vi "wherestheline.vi"(0 "SCin":u16=15000 min=10240 max=19650 step=100, 1 "S1in":u16=15000 min=10240 max=19650 step=100, 2 "S2in":u16=15000 min=10240 max=19650 step=100, 3 "S3in":u16=15000 min=10240 max=19650 step=100, 4 "S4in":u16=15000 min=10240 max=19650 step=100, 5 "S5in":u16=15000 min=10240 max=19650 step=100, 7 "last error":dbl=15000.0 min=10240.0 max=19650.0 step=100.0) -> (19 "SC":bool, 20 "error":dbl, 21 "line found":bool, 22 "really lost":bool, 23 "S1":bool, 24 "S2":bool, 25 "S3":bool, 26 "S4":bool, 27 "S5":bool)   [LabVIEW 2011]
panel:
  out "orS4":bool
  out "orS2":bool
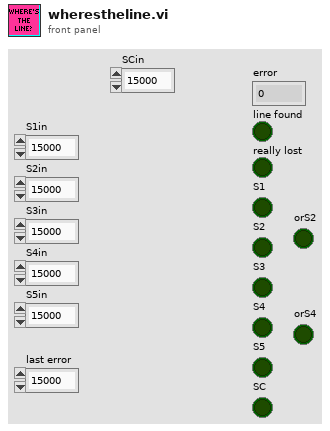
[diagram p1: front panel]
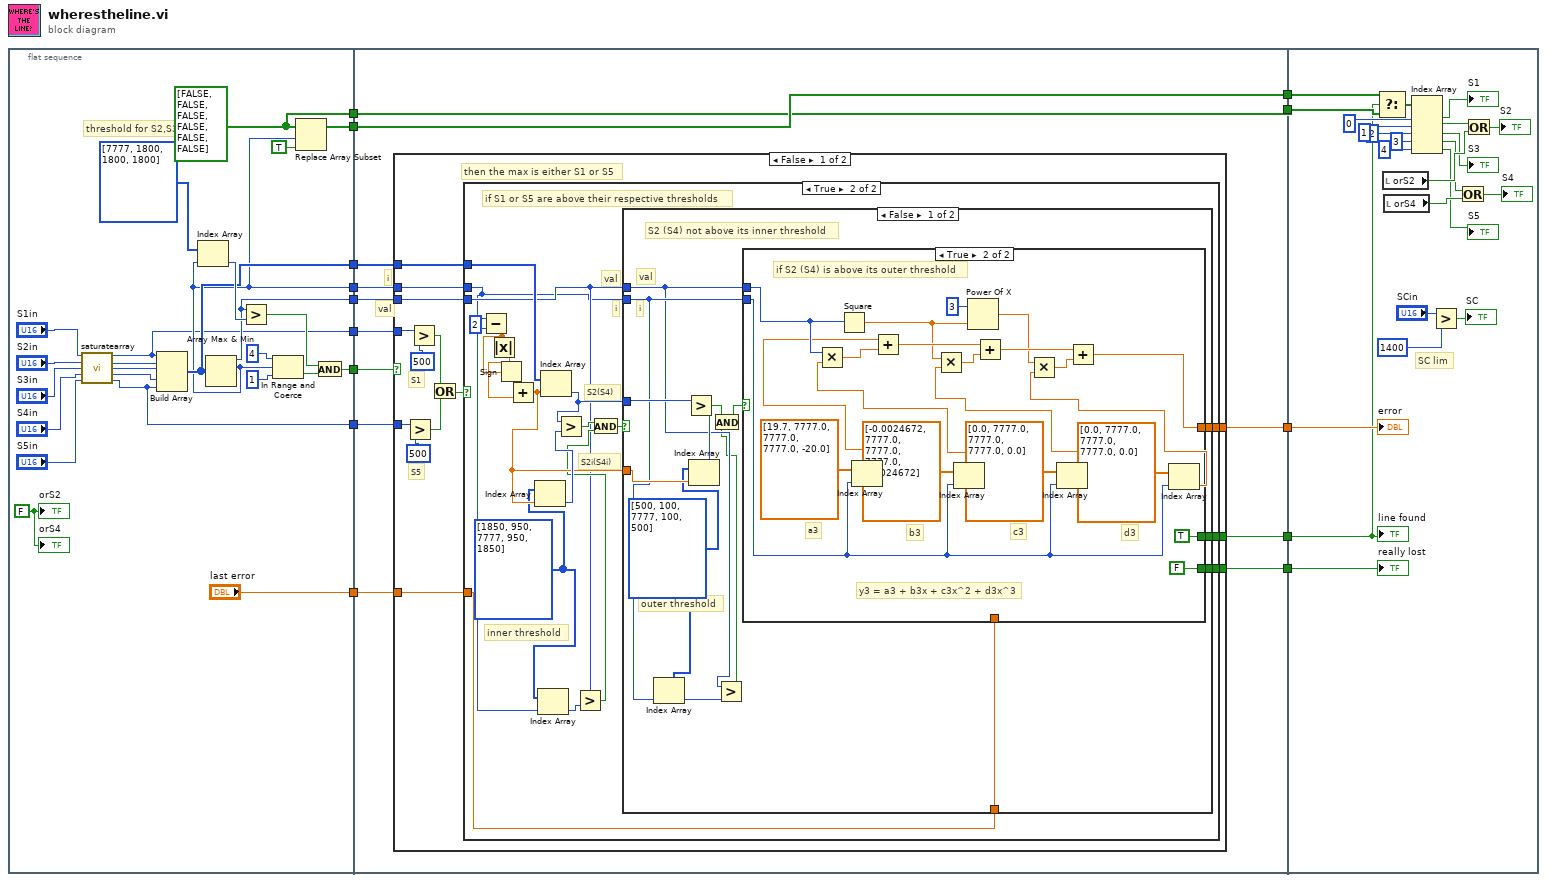
[diagram p0: block diagram]
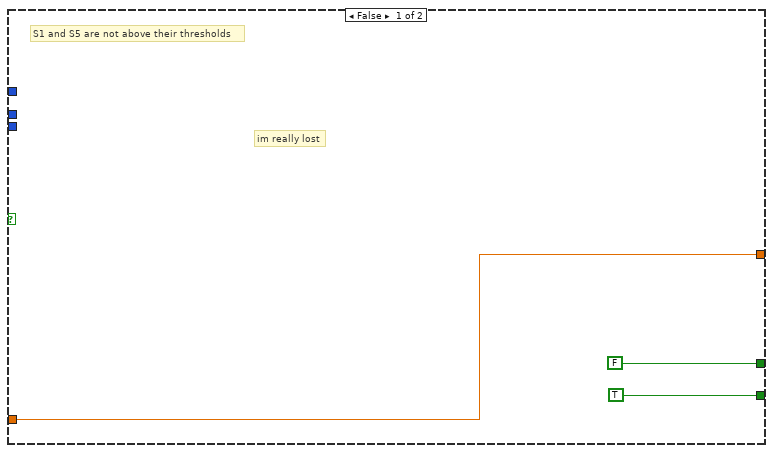
[diagram p2: hidden frame]
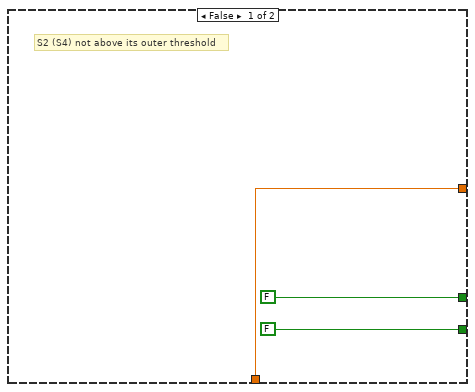
[diagram p3: hidden frame]
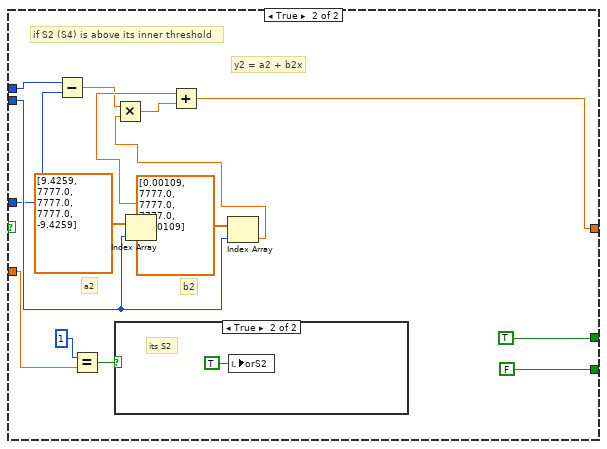
[diagram p4: hidden frame]
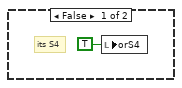
[diagram p5: hidden frame]
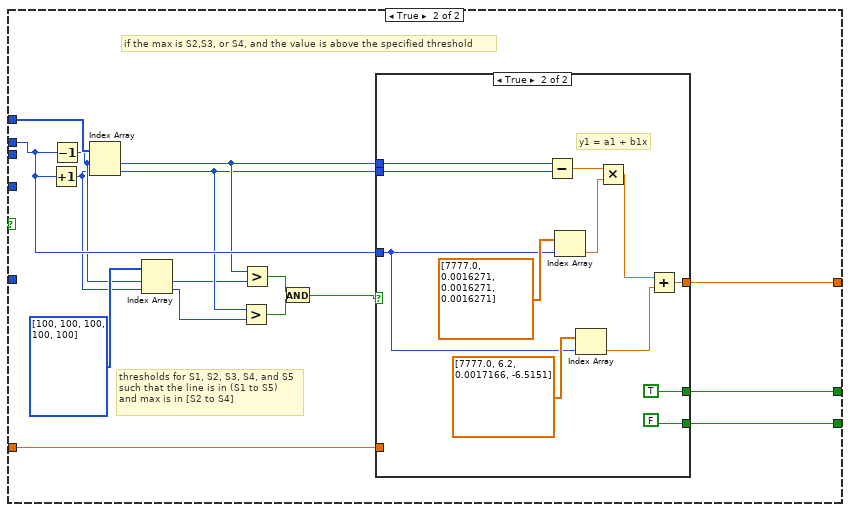
[diagram p6: hidden frame]
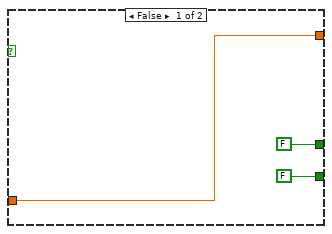
[diagram p7: hidden frame]
diagram:
  n1 = flat-sequence {
    tunnel: [w23] -> w14
    tunnel: [w22] -> w13
    tunnel: [w21] -> w12
    tunnel: [w20] -> w11
    tunnel: [w19] -> w10
    tunnel: [w18] -> w9
    tunnel: [w17] -> w8
    tunnel: [w16] -> w7
    tunnel: ["last error"] -> w6
    tunnel: w14 -> [w44]
    tunnel: w13 -> [w43]
    tunnel: w12 -> [w51]
    tunnel: w11 -> [w50]
    tunnel: w10 -> [w49]
    tunnel: w9 -> [w48]
    tunnel: w8 -> [w47]
    tunnel: w7 -> [w46]
    tunnel: w6 -> [w45]
    tunnel: [w44] -> w5
    tunnel: [w43] -> w4
    tunnel: [w42] -> w3
    tunnel: [w41] -> w2
    tunnel: [w40] -> w1
    tunnel: w5 -> [w179]
    tunnel: w4 -> [w178]
    tunnel: w3 -> [w177]
    tunnel: w2 -> [w176]
    tunnel: w1 -> [w175]
    frame #0 {
      w31 = FALSE ("orS2")
      w22 = bool[] [FALSE, FALSE, FALSE, FALSE, FALSE, FALSE]
      # "threshold for S2,S3,S4"
      n2 = call "saturatearray.vi"("S1in in"="S1in", "S2in in"="S2in", "S3in in"="S3in", "S4in in"="S4in", "S5in in"="S5in") -> ("S1in out"=w18:u16, "S2in out"=w32:u16, "S3in out"=w33:u16, "S4in out"=w34:u16, "S5in out"=w16:u16)  [unwired: 6 in]
      n3 = Build Array(w18, w32, w33, w34, w16) -> (w21:u16[])
      n4 = Array Max & Min(array=w21) -> (max value=w19:u16, max index (indices)=w20:i32)  [unwired: 2 out]
      n5 = Index Array(array=i32[] [7777, 1800, 1800, 1800], index=w20) -> (element=w29:i32)
      n6 = Greater?(x=w19, y=w29) -> (0:w28:bool)
      n7 = In Range and Coerce(upper limit=4, x=w20, lower limit=1) -> (In Range?=w27:bool)  [unwired: 1 out]
      n8 = Replace Array Subset(array=w22, new element=TRUE ("new element/subarray"), index=w20) -> (w23:bool[])
      n9 = And(x=w28, y=w27) -> (x .and. y?=w17:bool)
      "orS2" <- w31
      "orS4" <- w31
    }
    frame #1 {
      # "val"
      # "i"
      n10 = case shown="False" w47 {
        tunnel: w50 -> [w59 w154]
        tunnel: w51 -> [w58 w155]
        tunnel: w48 -> [w62 _]
        tunnel: w49 -> [w57 _]
        tunnel: [w56 w158] -> w42
        tunnel: [w54 w156] -> w41
        tunnel: w45 -> [w55 w143]
        tunnel: [w53 w157] -> w40
        tunnel: w46 -> [w52 _]
        frame False {
          # "S1"
          # "S5"
          # "then the max is either S1 or S5"
          n11 = Greater?(x=w52, y=u16 500) -> (0:w60:bool)
          n12 = Greater?(x=w62, y=u16 500) -> (0:w61:bool)
          n13 = Or(x=w61, y=w60) -> (x .or. y?=w65:bool)
          n14 = case shown="True" w65 {
            tunnel: w59 -> [_ w70]
            tunnel: w58 -> [_ w83]
            tunnel: w57 -> [_ w71]
            tunnel: [w68 w82] -> w56
            tunnel: w55 -> [w68 w80]
            tunnel: [FALSE w81] -> w54
            tunnel: [TRUE w79] -> w53
            frame False {
              # "im really lost"
              # "S1 and S5 are not above their thresholds"
            }
            frame True {
              w76 = i32[] [1850, 950, 7777, 950, 1850]
              # "i"
              # "val"
              # "S2(S4)"
              # "S2i(S4i)"
              # "inner threshold"
              # "if S1 or S5 are above their respective thresholds"
              n15 = Subtract(x=w70, y=2) -> (x-y=w78:dbl)
              n16 = Absolute Value(x=w78) -> (abs(x)=w77:dbl)
              n17 = Sign(1:w78) -> (0:w87:dbl)
              n18 = Add(x=w87, y=w77) -> (x+y=w84:dbl)
              n19 = Index Array(array=w76, index=w84) -> (element=w86:i32)
              n20 = Index Array(array=w76, index=w70) -> (element=w75:i32)
              n21 = Index Array(array=w83, index=w84) -> (element=w85:u16)
              n22 = Greater?(x=w85, y=w86) -> (0:w73:bool)
              n23 = Greater?(x=w71, y=w75) -> (0:w72:bool)
              n24 = And(x=w73, y=w72) -> (x .and. y?=w74:bool)
              n25 = case shown="False" w74 {
                tunnel: w85 -> [w101 w126]
                tunnel: w84 -> [w100 w132]
                tunnel: w71 -> [w91 w128]
                tunnel: w70 -> [w93 w136]
                tunnel: [w98 w129] -> w82
                tunnel: [w97 TRUE] -> w81
                tunnel: w80 -> [w96 _]
                tunnel: [w95 FALSE] -> w79
                frame False {
                  w94 = i32[] [500, 100, 7777, 100, 500]
                  # "val"
                  # "i"
                  # "S2 (S4) not above its inner threshold"
                  # "outer threshold"
                  n26 = Index Array(array=w94, index=w93) -> (element=w92:i32)
                  n27 = Index Array(array=w94, index=w100) -> (element=w99:i32)
                  n28 = Greater?(x=w101, y=w99) -> (0:w89:bool)
                  n29 = Greater?(x=w91, y=w92) -> (0:w88:bool)
                  n30 = And(x=w89, y=w88) -> (x .and. y?=w90:bool)
                  n31 = case shown="True" w90 {
                    tunnel: w91 -> [_ w109]
                    tunnel: w93 -> [_ w110]
                    tunnel: [w103 w108] -> w98
                    tunnel: [FALSE TRUE] -> w97
                    tunnel: w96 -> [w103 _]
                    tunnel: [FALSE FALSE] -> w95
                    frame False {
                      # "S2 (S4) not above its outer threshold"
                    }
                    frame True {
                      # "d3"
                      # "c3"
                      # "b3"
                      # "a3"
                      # "y3 = a3 + b3x + c3x^2 + d3x^3"
                      # "if S2 (S4) is above its outer threshold"
                      n32 = Square(x=w109) -> (x^2=w114:dbl)
                      n33 = Index Array(array=dbl[] [19.7, 7777.0, 7777.0, 7777.0, -20.0], index=w110) -> (element=w105:dbl)
                      n34 = Index Array(array=dbl[] [-0.0024672, 7777.0, 7777.0, 7777.0, 0.0024672], index=w110) -> (element=w121:dbl)
                      n35 = Multiply(x=w109, y=w121) -> (x*y=w122:dbl)
                      n36 = Add(x=w105, y=w122) -> (x+y=w119:dbl)
                      n37 = Power Of X(1:w114, 2:3 ("y")) -> (0:w112:dbl)
                      n38 = Index Array(array=dbl[] [0.0, 7777.0, 7777.0, 7777.0, 0.0], index=w110) -> (element=w120:dbl)
                      n39 = Multiply(x=w114, y=w120) -> (x*y=w118:dbl)
                      n40 = Add(x=w119, y=w118) -> (x+y=w115:dbl)
                      n41 = Index Array(array=dbl[] [0.0, 7777.0, 7777.0, 7777.0, 0.0], index=w110) -> (element=w111:dbl)
                      n42 = Multiply(x=w112, y=w111) -> (x*y=w116:dbl)
                      n43 = Add(x=w115, y=w116) -> (x+y=w108:dbl)
                    }
                  }
                }
                frame True {
                  # "b2"
                  # "a2"
                  # "y2 = a2 + b2x"
                  # "if S2 (S4) is above its inner threshold"
                  n44 = Subtract(x=w128, y=w126) -> (x-y=w127:dbl)
                  n45 = Equal?(x=u16 1 ("t"), y=w132) -> (x = y?=w131:bool)
                  n46 = case shown="True" w131 {
                    frame False {
                      # "its S4"
                      n47 = local write "orS4"(TRUE ("orS2")) -> ()
                    }
                    frame True {
                      # "its S2"
                      n48 = local write "orS2"(TRUE ("orS2")) -> ()
                    }
                  }
                  n49 = Index Array(array=dbl[] [9.4259, 7777.0, 7777.0, 7777.0, -9.4259], index=w136) -> (element=w130:dbl)
                  n50 = Index Array(array=dbl[] [0.00109, 7777.0, 7777.0, 7777.0, -0.00109], index=w136) -> (element=w137:dbl)
                  n51 = Multiply(x=w127, y=w137) -> (x*y=w138:dbl)
                  n52 = Add(x=w130, y=w138) -> (x+y=w129:dbl)
                }
              }
            }
          }
        }
        frame True {
          # "thresholds for S1, S2, S3, S4, and S5\nsuch that the line is in (S1 to S5)\nand max is in [S2 to S4]"
          # "if the max is S2,S3, or S4, and the value is above the specified threshold"
          n53 = Increment(x=w154) -> (x+1=w150:i32)
          n54 = Decrement(x=w154) -> (x-1=w151:i32)
          n55 = Index Array(array=w155, index #1=w151, index #2=w150) -> (element #1=w153:u16, element #2=w149:u16)
          n56 = Index Array(array=i32[] [100, 100, 100, 100, 100], index #1=w151, index #2=w150) -> (element #1=w148:i32, element #2=w147:i32)
          n57 = Greater?(x=w149, y=w147) -> (0:w145:bool)
          n58 = Greater?(x=w153, y=w148) -> (0:w146:bool)
          n59 = And(x=w146, y=w145) -> (x .and. y?=w144:bool)
          n60 = case shown="True" w144 {
            tunnel: [w159 w168] -> w158
            tunnel: [FALSE ("new element/subarray") FALSE] -> w157
            tunnel: [FALSE ("new element/subarray") TRUE] -> w156
            tunnel: w153 -> [_ w164]
            tunnel: w149 -> [_ w163]
            tunnel: w154 -> [_ w162]
            tunnel: w143 -> [w159 _]
            frame False {
            }
            frame True {
              # "y1 = a1 + b1x"
              # "b1"
              # "a1"
              n61 = Subtract(x=w164, y=w163) -> (x-y=w165:dbl)
              n62 = Index Array(array=dbl[] [7777.0, 0.0016271, 0.0016271, 0.0016271], index=w162) -> (element=w171:dbl)
              n63 = Index Array(array=dbl[] [7777.0, 6.2, 0.0017166, -6.5151], index=w162) -> (element=w170:dbl)
              n64 = Multiply(x=w165, y=w171) -> (x*y=w169:dbl)
              n65 = Add(x=w169, y=w170) -> (x+y=w168:dbl)
            }
          }
        }
      }
    }
    frame #2 {
      # "SC lim"
      n66 = Select(t=w179, s=w176, f=w178) -> (s? t:f=w180:bool[])
      n67 = local read "orS2"() -> (w193:bool)
      n68 = local read "orS4"() -> (w194:bool)
      n69 = Index Array(array=w180, index #1=0 ("index"), index #2=1 ("index"), index #3=2 ("index"), index #4=3 ("index"), index #5=4 ("index")) -> (element #1=→"S1":bool, element #2=w191:bool, element #3=→"S3":bool, element #4=w189:bool, element #5=→"S5":bool)
      n70 = Greater?(x="SCin", y=u16 1400) -> (0:→"SC":bool)
      n71 = Or(x=w189, y=w194) -> (x .or. y?=→"S4":bool)
      n72 = Or(x=w191, y=w193) -> (x .or. y?=→"S2":bool)
      "error" <- w177
      "line found" <- w176
      "really lost" <- w175
    }
  }
